vi "Set Tasks.vi"(8 "error in (no error)":errorcluster, 10 "Tasks":map{string, refnum<class "Task Base.lvclass">}(c390), 11 "HAL GOOP4:Series Base in":refnum<class "Series Base.lvclass">) -> (0 "error out":errorcluster, 3 "HAL GOOP4:Series Base out":refnum<class "Series Base.lvclass">)   [LabVIEW 2023, in "HAL GOOP4.lvlib" / "Series Base.lvclass"]
uses:
  Series Base.lvclass
  Task/Task Base/Task Base.lvclass
  Series Base.lvclass/Series Base.ctl
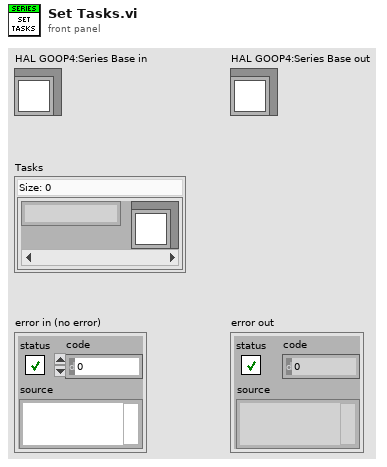
[diagram p1: front panel]
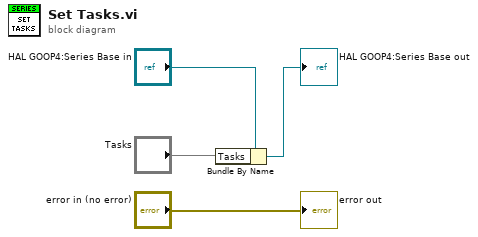
[diagram p0: block diagram]
diagram:
  n1 = Bundle By Name(cluster="HAL GOOP4:Series Base in", "Tasks"="Tasks") -> (→"HAL GOOP4:Series Base out":refnum<class "Series Base.lvclass">)
  "error out" <- "error in (no error)"
